vi "BK7 Test Scanner.vi"() -> ()   [LabVIEW 2016]
uses:
  <vilib>/vision/Image Controls.llb/IMAQ Image.ctl
  Hardware Configuration/Hardware Configuration Controls/Device Type.ctl
  Hardware Configuration/Hardware Configuration Controls/Device Function.ctl
  Device Library/Cameras/Hamamatsu/Orca Flash/Orca Flash Controls/Orca Flash Actions.ctl
  Device Library/Cameras/Camera Controls/Camera IMAQ Key Info.ctl
  Display Module/Display Module Custom Controls/ROI Descriptor.ctl
  <vilib>/vision/NI_Vision_Development_Module.lvlib
panel:
  out "Mean Value":sgl(graph)
  out "Max Value":sgl(graph)
  in  "stop":bool
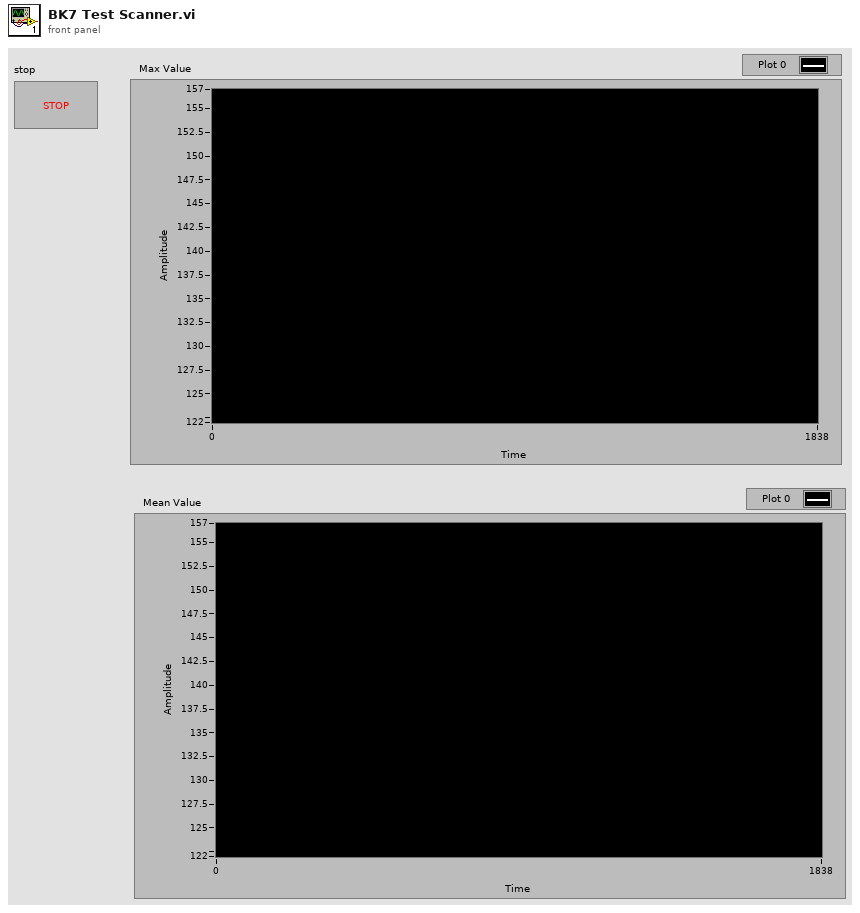
[diagram p1: front panel]
types:
  T1 = typedef "Image Type" = u32
  T2 = typedef "Orca Flash Actions.ctl" = enum16{"IDLE", "PREVIEW", "RECORD", "Record Settings", "SETPARAM", "GETPARAM", "SETROI", "GETROI", "PROGRESSIVE MODE", "AREA MODE", "STATUS", "QUIT"}
  T3 = typedef "Device Function.ctl" = enum16{"Primary", "Secondary", "Overview", "Wide Field Drift Correction", "642 nm Excitation", "560 nm Excitation", "546 nm Excitation", "488 nm Excitation", "405 nm Excitation", "Objective Drift Correction", "Objective XY", "Objective Z", "Sample XY", "Sample Coarse Z", "Sample Z", "4Pi Lower", "4Pi Upper", "Adj Cavity"}
  T4 = typedef "Device Type.ctl" = enum16{"AOTF", "Camera", "Deformable Mirror", "Laser", "Shutter", "Stage"}
  T5 = typedef "IMAQ Image.ctl" = refnum<image>
  T6 = typedef "ROI Descriptor.ctl" = cluster{"Global Rectangle":i32[], "Contours":cluster{"Contour Type":u32, "ROI Type":u32, "Points":i32[]}[]}
  T7 = typedef "Camera IMAQ Key Info.ctl" = cluster{"Frame":u32, "Sensor Height":i32, "Sensor Width":i32, "ROI Height":i32, "ROI Width":i32, "ROI Enable?":bool, "Bit per Pixel":u8}
  T8 = cluster{"Mean Value":sgl, "Standard Variation":sgl, "Minimal Value":sgl, "Maximal Value":sgl, "Area (calibrated)":sgl, "Area (pixels)":u32, "%":sgl, "Calibration Valid":bool}
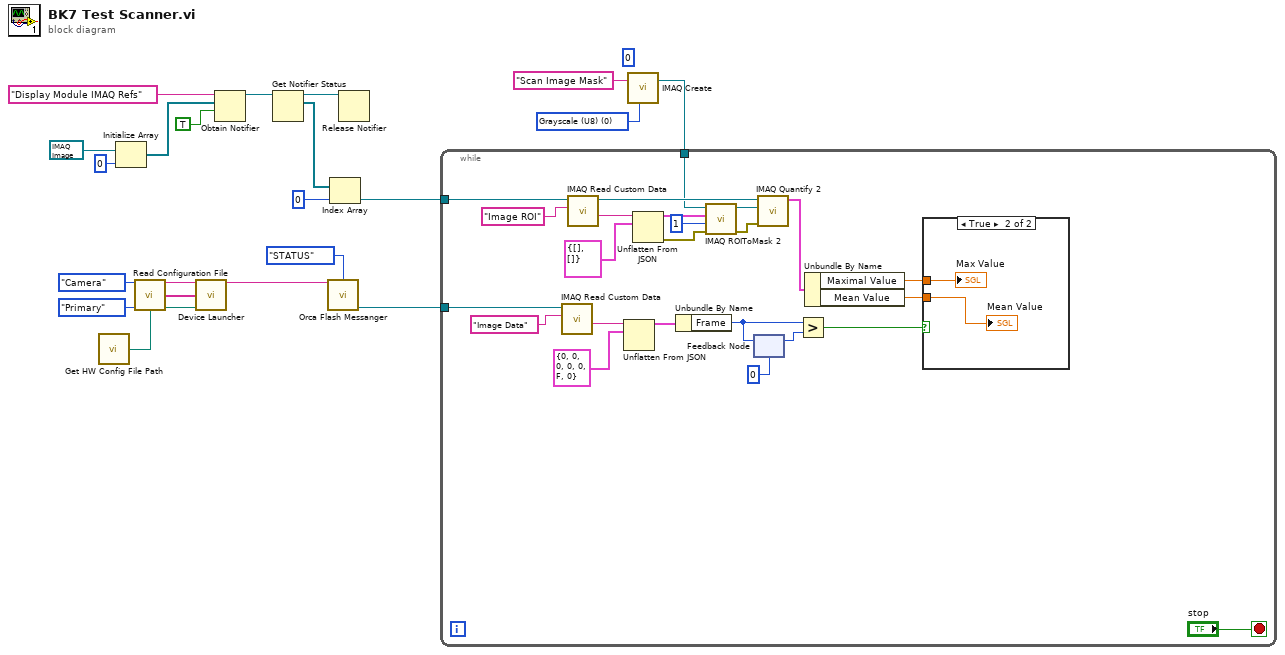
[diagram p0: block diagram]
diagram:
  w2 = T1 0 items=["Grayscale (U8)", "Grayscale (I16)", "Grayscale (SGL)", "Complex (CSG)", "RGB (U32)", "HSL (U32)", "RGB (U64)", "Grayscale (U16)"] ("Image Type")
  (unwired) 0 ("Border Size")
  n1 = call "Get HW Config File Path.vi"() -> ("File Path"=w9:path)  [unwired: 14 in, 1 out]
  n2 = Initialize Array(T5 refnum ("New Image"), 0 ("dimension size")) -> (w18:T5[])
  n3 = call "Read Configuration File.vi"("Device Type"=Device_Type."Camera", "Device Function"=Device_Function."Primary", "Config File Path"=w9) -> ("Unique Notifier Name"=w10:string, "Device Ports/IDs/Channels"=w12:string[], "Device Engine Path"=w11:path)  [unwired: 9 in, 1 out]
  n4 = call "Device Launcher.vi"("Notifier Name"=w10, "Device Ports/IDs/Channels"=w12, "Device Engine Path"=w11) -> ("Notifier Name"=w6:string)  [unwired: 11 in, 1 out]
  n5 = Obtain Notifier(name (unnamed)="Display Module IMAQ Refs", notification data type=w18, create if not found? (T)=TRUE) -> (notifier out=w17:refnum<notifier>)  [unwired: 1 in, 2 out]
  n6 = Get Notifier Status(notifier=w17) -> (notifier out=w8:refnum<notifier>, current notification=w16:T5[])  [unwired: 1 in, 3 out]
  n7 = call "Orca Flash Messanger.vi"("Notifier Name"=w6, "Camera Actions"=Orca_Flash_Actions."STATUS") -> ("Image Ref"=w4:T5)  [unwired: 9 in, 4 out]
  n8 = Index Array(array=w16, index=0) -> (element=w5:T5)
  n9 = Release Notifier(notifier=w8) -> ()  [unwired: 2 in, 3 out]
  n10 = call "IMAQ Create"("Image Name"="Scan Image Mask", "Image Type"=w2) -> ("New Image"=w1:T5)  [unwired: 3 in, 1 out]
  n11 = while {
    tunnel: w5 -> [w27]
    tunnel: w4 -> [w38]
    tunnel: w1 -> [w26]
    stop <- "stop" stop-if-true
    n12 = call "IMAQ Read Custom Data"("Key"="Image Data", "Image"=w38) -> ("Custom Data Out"=w44:string)  [unwired: 7 in, 2 out]
    n13 = call "IMAQ Read Custom Data"("Key"="Image ROI", "Image"=w27) -> ("Custom Data Out"=w36:string, "Image (duplicate)"=w28:T5)  [unwired: 7 in, 1 out]
    n14 = Unflatten From JSON(JSON string=w44, type and defaults=T7 {"Frame"=0, "Sensor Height"=0, "Sensor Width"=0, "ROI Height"=0, "ROI Width"=0, "ROI Enable?"=FALSE, "Bit per Pixel"=0} ("Camera IMAQ Key Info")) -> (value=w42:T7)  [unwired: 5 in, 1 out]
    n15 = Unflatten From JSON(JSON string=w36, type and defaults=T6 {"Global Rectangle"=[], "Contours"=[]} ("Image ROI Descriptor")) -> (value=w34:T6, error out=w30:errorcluster)  [unwired: 5 in]
    n16 = Unbundle By Name(w42) -> ("Frame"=w41:u32)
    n17 = call "IMAQ ROIToMask 2"("error in (no error)"=w30, "Filling Value (255)"=1, "ROI Descriptor"=w34, "Image"=w26) -> ("error out"=w31:errorcluster, "Image Out"=w32:T5)  [unwired: 5 in, 1 out]
    n18 = feedback #1(u32 0 ("Frame")) -> (w40:u32)
    n19 = feedback-in #1(w41) -> ()
    n20 = call "IMAQ Quantify 2"("error in (no error)"=w31, "Image Mask"=w32, "Image"=w28) -> ("Global Report"=w29:T8)  [unwired: 6 in, 2 out]
    n21 = Greater?(x=w41, y=w40) -> (0:w25:bool)
    n22 = Unbundle By Name(w29) -> ("Maximal Value"=w24:sgl, "Mean Value"=w23:sgl)
    n23 = case shown="True" w25 {
      tunnel: w24 -> [_ w48]
      tunnel: w23 -> [_ w47]
      frame False {
      }
      frame True {
        "Max Value" <- w48
        "Mean Value" <- w47
      }
    }
  }
